vi "Front panel phase out.vi"(6 "close?":bool=TRUE, 7 "Mode":enum16{"In", "Out"}(ring), 8 "error in (no error)":errorcluster, 9 "millisecond multiple out":u32=10, 10 "millisecond multiple In":u32=10, 11 "path":path) -> (0 "error out":errorcluster)   [LabVIEW 2016]
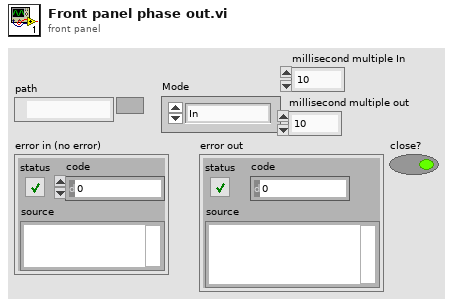
[diagram p1: front panel]
types:
  T1 = enum32{"Invalid", "Standard", "Closed", "Hidden", "Minimized", "Maximized"}
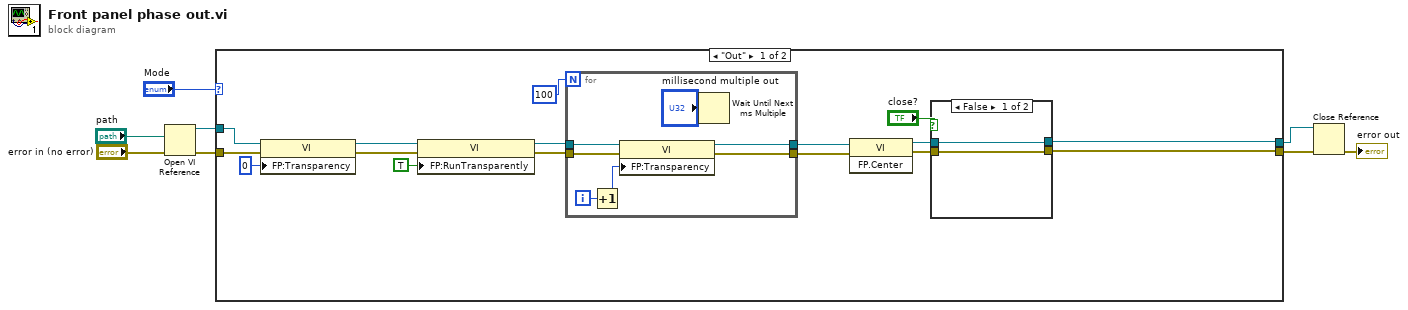
[diagram p0: block diagram]
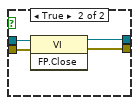
[diagram p2: hidden frame]
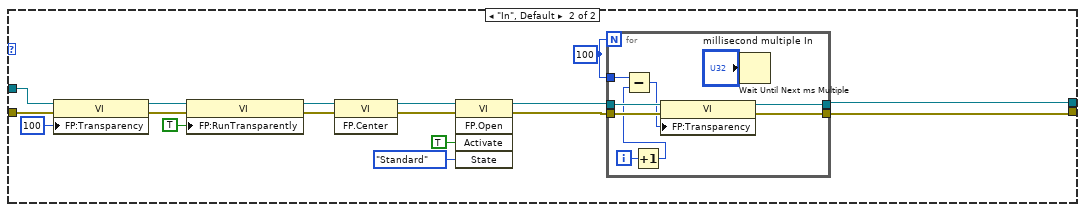
[diagram p3: hidden frame]
diagram:
  n1 = Open VI Reference(vi path="path", error in (no error)="error in (no error)") -> (vi reference=w5:refnum<vi>, error out=w6:errorcluster)  [unwired: 4 in]
  n2 = case shown="\"Out\"" "Mode" {
    tunnel: w6 -> [w18 w53]
    tunnel: w5 -> [w14 w49]
    tunnel: [w10 w45] -> w4
    tunnel: [w11 w44] -> w3
    frame "Out" {
      n3 = property class="VI"(reference=w14, error in=w18, "FP:Transparency"=u8 0 ("Front Panel Window:Transparency")) -> (reference out=w15:refnum<vi>, error out=w17:errorcluster)
      n4 = property class="VI"(reference=w15, error in=w17, "FP:RunTransparently"=TRUE ("Front Panel Window:Run VI Transparently")) -> (reference out=w19:refnum<vi>, error out=w20:errorcluster)
      n5 = for {
        N: 100 -> [_]
        tunnel: w19 -> [w37]
        tunnel: w20 -> [w36]
        tunnel: [w35] -> w24
        tunnel: [w34] -> w23
        i -> [w32]
        n6 = Increment(x=w32) -> (x+1=w31:i32)
        n7 = property class="VI"(reference=w37, error in=w36, "FP:Transparency"=w31) -> (reference out=w34:refnum<vi>, error out=w35:errorcluster)
        n8 = Wait Until Next ms Multiple(millisecond multiple="millisecond multiple out") -> ()  [unwired: 1 out]
      }
      n9 = invoke class="VI" method="FP.Center"(reference=w23, error in=w24) -> (reference out=w12:refnum<vi>, error out=w13:errorcluster)  [unwired: 1 in, 1 out]
      n10 = case shown="False" "close?" {
        tunnel: w13 -> [w26 w30]
        tunnel: w12 -> [w25 w29]
        tunnel: [w25 w28] -> w11
        tunnel: [w26 w27] -> w10
        frame False {
        }
        frame True {
          n11 = invoke class="VI" method="FP.Close"(reference=w29, error in=w30) -> (reference out=w28:refnum<vi>, error out=w27:errorcluster)  [unwired: 1 in, 1 out]
        }
      }
    }
    frame "In", Default {
      w48 = 100
      n12 = property class="VI"(reference=w49, error in=w53, "FP:Transparency"=u8 100 ("Front Panel Window:Transparency")) -> (reference out=w50:refnum<vi>, error out=w52:errorcluster)
      n13 = property class="VI"(reference=w50, error in=w52, "FP:RunTransparently"=TRUE ("Front Panel Window:Run VI Transparently")) -> (reference out=w46:refnum<vi>, error out=w47:errorcluster)
      n14 = invoke class="VI" method="FP.Center"(reference=w46, error in=w47) -> (reference out=w43:refnum<vi>, error out=w42:errorcluster)  [unwired: 1 in, 1 out]
      n15 = invoke class="VI" method="FP.Open"(reference=w43, error in=w42, "Activate"=TRUE ("Activate?"), "State"=T1."Standard") -> (reference out=w41:refnum<vi>, error out=w40:errorcluster)  [unwired: 1 in, 3 out]
      n16 = for {
        N: w48 -> [_]
        tunnel: w41 -> [w63]
        tunnel: w40 -> [w62]
        tunnel: [w61] -> w45
        tunnel: [w60] -> w44
        tunnel: w48 -> [w57]
        i -> [w58]
        n17 = Increment(x=w58) -> (x+1=w56:i32)
        n18 = Subtract(x=w57, y=w56) -> (x-y=w55:i32)
        n19 = property class="VI"(reference=w63, error in=w62, "FP:Transparency"=w55) -> (reference out=w60:refnum<vi>, error out=w61:errorcluster)
        n20 = Wait Until Next ms Multiple(millisecond multiple="millisecond multiple In") -> ()  [unwired: 1 out]
      }
    }
  }
  n21 = Close Reference(reference=w3, error in (no error)=w4) -> (error out=→"error out":errorcluster)
